vi "Memory.Pointer.Numeric.Set power of 2.vi"(8 "error in (no error)":errorcluster, 10 "power of 2":i16, 11 "Numeric Pointer in":refnum<class "Memory.Pointer.Numeric.lvclass">) -> (0 "error out":errorcluster, 3 "Numeric Pointer out":refnum<class "Memory.Pointer.Numeric.lvclass">)   [LabVIEW 2016, in "Memory.Pointer.Numeric.lvclass"]
uses:
  Memory.Pointer.Numeric.lvclass
  C:/Users/Ryan/Documents/Git/Sourcetree/LabVIEW-Memory-Manager/Source/Library/Classes/Pointer/Pointer.Void/Memory.Pointer.Void.lvclass
  Memory.Pointer.Numeric.lvclass/Memory.Pointer.Numeric.ctl
  Pointer.Void/Memory.Pointer.Void.lvclass/Memory.Pointer.Void.ctl
  Pointer.Void/Memory.Pointer.Void.lvclass
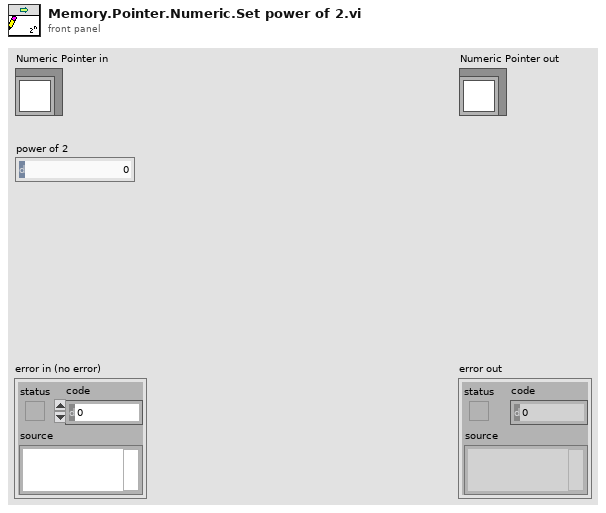
[diagram p1: front panel]
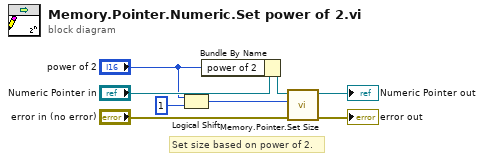
[diagram p0: block diagram]
diagram:
  # "Set size based on power of 2."
  n1 = Logical Shift(y="power of 2", x=u64 1) -> (x << y=w7:u64)
  n2 = Bundle By Name(cluster="Numeric Pointer in", "power of 2"="power of 2") -> (w2:refnum<class "Memory.Pointer.Numeric.lvclass">)
  n3 = call "Memory.Pointer.Set Size.vi"("error in (no error)"="error in (no error)", "size"=w7, "Pointer in"=w2) -> ("error out"=→"error out":errorcluster, "Pointer out"=→"Numeric Pointer out":refnum<class "Memory.Pointer.Numeric.lvclass">)  [unwired: 7 in]
